vi "Main.vi"   [LabVIEW 2016]
uses:
  server/server/server.lvclass
  C:/Program Files/National Instruments/LabVIEW 2016/vi.lib/ActorFramework/Actor/Actor.lvclass
  <vilib>/ActorFramework/Actor/Actor.lvclass
panel:
  # "Launch Actor---Main()"
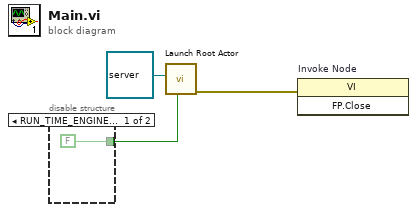
[diagram p0: block diagram]
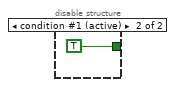
[diagram p2: hidden frame]
diagram:
  n1 = disable-structure shown="RUN_TIME_ENGINE==True" {
    disable-tunnel: [FALSE TRUE ("Open Actor Core front panel? (F)")] -> w1
    frame condition #0 {
    }
    frame condition #1 (active) {
    }
  }
  n2 = call <vilib>:"Launch Root Actor.vi"("Open Actor Core front panel? (F)"=w1, "Actor"=refnum<class "server.lvclass"> refnum ("server.lvlib:server.lvclass")) -> ("error out"=w2:errorcluster)  [unwired: 8 in, 1 out]
  n3 = invoke on="Invoke Node" class="VI" method="FP.Close"(error in=w2) -> ()  [unwired: 2 in, 3 out]
